vi "ith Field.vi"(0 "ith step":u16, 1 "RampParameter":dbl[](array[numeric])=[0.0, 30.0, 1.0, 20.0] format="%.2f", 3 "Maximum Allowed Current":dbl=100.0 format="%.2f", 4 "stopCycle":bool) -> (5 "Goto Field":dbl format="%.2f", 6 "Ramp Speed":dbl=20.0 format="%.2f", 7 "Stop?":bool=TRUE)   [LabVIEW 2025]
doc: "This Vi extract current field and set the scan continue boolean variable.\n\nThe field step can be either positive or negative.\n\nIf any of the absolute field value exceeds the maximum allowed limit, it will be replaced with the maximum field value itself\nAuthor: Scott Hannahs <sth@magnet.fsu.edu>\n\nThis software is licensed for use under the “MIT License\"\nCopyright (c) 2025 Scott Hannahs, sth@sth@magnet.sthnet.net\n\nPermission is hereby granted, free of charge, to any person obtaining a copy of this software and associated documentation files (the \"Software\"), to deal in the Software without restriction, including without limitation the rights to use, copy, modify, merge, publish, distribute, sublicense, and/or sell copies of the Software, and to permit persons to whom the Software is furnished to do so, subject to the following conditions: The above copyright notice and this permission notice shall be included in all copies or substantial portions of the Software.\n\nTHE SOFTWARE IS PROVIDED \"AS IS\", WITHOUT WARRANTY OF ANY KIND, EXPRESS OR IMPLIED, INCLUDING BUT NOT LIMITED TO THE WARRANTIES OF MERCHANTABILITY, FITNESS FOR A PARTICULAR PURPOSE AND NONINFRINGEMENT. IN NO EVENT SHALL THE AUTHORS OR COPYRIGHT HOLDERS BE LIABLE FOR ANY CLAIM, DAMAGES OR OTHER LIABILITY, WHETHER IN AN ACTION OF CONTRACT, TORT OR OTHERWISE, ARISING FROM, OUT OF OR IN CONNECTION WITH THE SOFTWARE OR THE USE OR OTHER DEALINGS IN THE SOFTWARE."
panel:
  out "Field Step":dbl=0.5 format="%.2f"
  out "Final Field":dbl=45.0 format="%.2f"
  out "Initial Field":dbl format="%.2f"
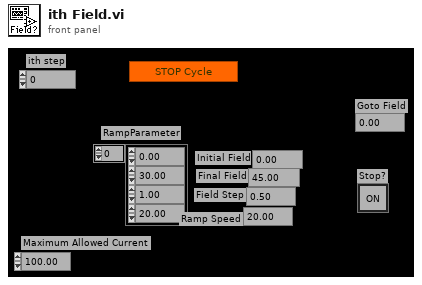
[diagram p1: front panel]
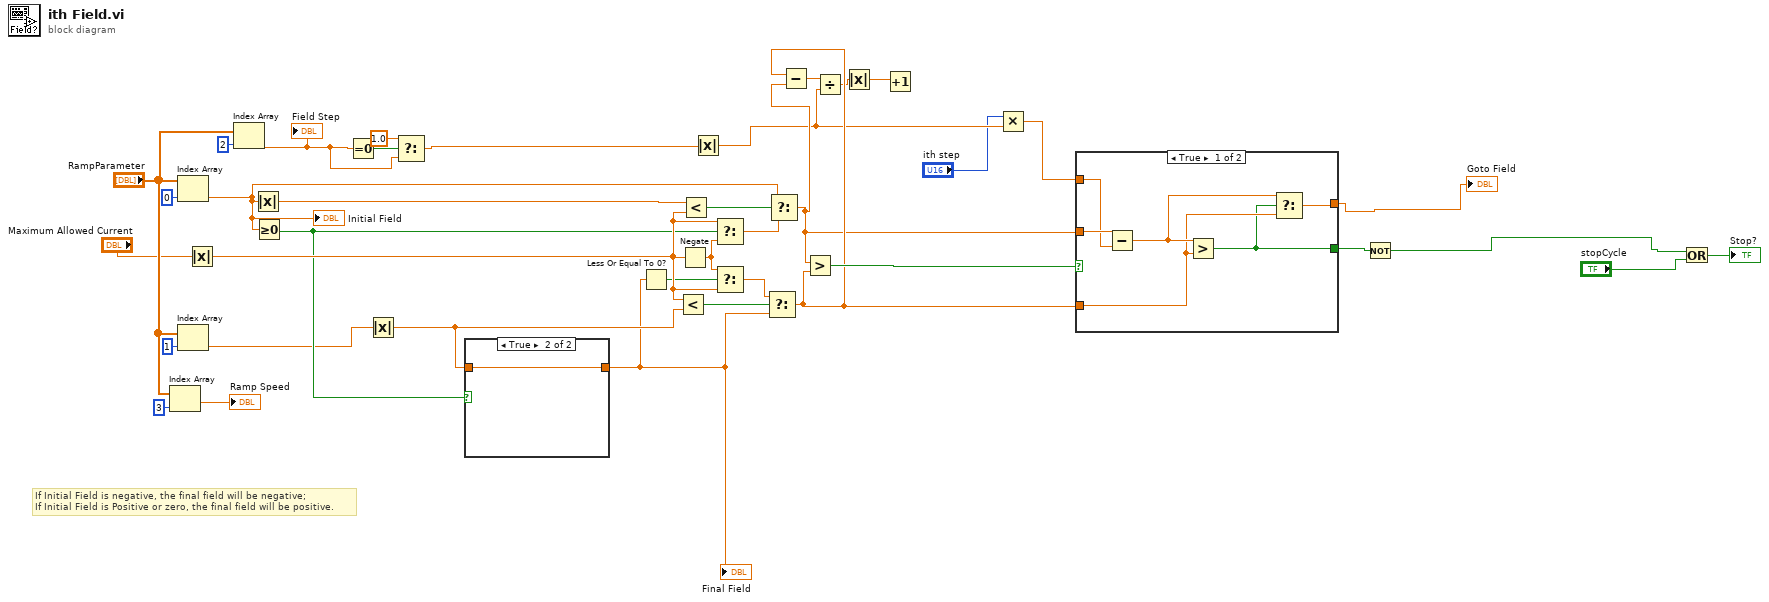
[diagram p0: block diagram]
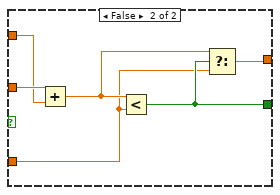
[diagram p2: hidden frame]
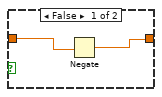
[diagram p3: hidden frame]
diagram:
  # "If Initial Field is negative, the final field will be negative;\nIf Initial Field is Positive or zero, the final field will be positive."
  n1 = Index Array(array="RampParameter", index=3) -> (element=→"Ramp Speed":dbl)
  n2 = Index Array(array="RampParameter", index=0) -> (element=w30:dbl)
  "Initial Field" <- w30
  n3 = Index Array(array="RampParameter", index=1) -> (element=w26:dbl)
  n4 = Absolute Value(x="Maximum Allowed Current") -> (abs(x)=w36:dbl)
  n5 = Index Array(array="RampParameter", index=2) -> (element=w22:dbl)
  "Field Step" <- w22
  n6 = Absolute Value(x=w30) -> (abs(x)=w37:dbl)
  n7 = Greater Or Equal To 0?(x=w30) -> (x >= 0?=w28:bool)
  n8 = Equal To 0?(x=w22) -> (x = 0?=w23:bool)
  n9 = Absolute Value(x=w26) -> (abs(x)=w27:dbl)
  n10 = Select(t=1.0, s=w23, f=w22) -> (s? t:f=w20:dbl)
  n11 = case shown="True" w28 {
    tunnel: w27 -> [w40 w41]
    tunnel: [w39 w41] -> w25
    frame False {
      n12 = Negate(x=w40) -> (-x=w39:dbl)
    }
    frame True {
    }
  }
  "Final Field" <- w25
  n13 = Less Or Equal To 0?(x=w25) -> (x <= 0?=w15:bool)
  n14 = Less?(x=w36, y=w27) -> (x < y?=w17:bool)
  n15 = Negate(x=w36) -> (-x=w14:dbl)
  n16 = Less?(x=w37, y=w36) -> (x < y?=w18:bool)
  n17 = Absolute Value(x=w20) -> (abs(x)=w9:dbl)
  n18 = Select(t=w36, s=w28, f=w14) -> (s? t:f=w16:dbl)
  n19 = Select(t=w14, s=w15, f=w36) -> (s? t:f=w13:dbl)
  n20 = Select(t=w13, s=w17, f=w25) -> (s? t:f=w12:dbl)
  n21 = Select(t=w30, s=w18, f=w16) -> (s? t:f=w11:dbl)
  n22 = Subtract(x=w12, y=w11) -> (x-y=w10:dbl)
  n23 = Greater?(x=w11, y=w12) -> (0:w19:bool)
  n24 = Divide(x=w10, y=w9) -> (x/y=w8:dbl)
  n25 = Absolute Value(x=w8) -> (abs(x)=w7:dbl)
  n26 = Increment(x=w7) -> ()  [unwired: 1 out]
  n27 = Multiply(x="ith step", y=w9) -> (x*y=w6:dbl)
  n28 = case shown="True" w19 {
    tunnel: [w42 w50] -> w3
    tunnel: w11 -> [w47 w53]
    tunnel: w12 -> [w43 w49]
    tunnel: w6 -> [w46 w52]
    tunnel: [w45 w48] -> w5
    frame True {
      n29 = Subtract(x=w47, y=w46) -> (x-y=w44:dbl)
      n30 = Greater?(x=w44, y=w43) -> (0:w42:bool)
      n31 = Select(t=w44, s=w42, f=w43) -> (s? t:f=w45:dbl)
    }
    frame False {
      n32 = Add(x=w53, y=w52) -> (x+y=w51:dbl)
      n33 = Less?(x=w51, y=w49) -> (x < y?=w50:bool)
      n34 = Select(t=w51, s=w50, f=w49) -> (s? t:f=w48:dbl)
    }
  }
  "Goto Field" <- w5
  n35 = Not(x=w3) -> (.not. x?=w2:bool)
  n36 = Or(x=w2, y="stopCycle") -> (x .or. y?=→"Stop?":bool)
